vi "Save spectrum data.vi"(9 "Sample Temperature Unit":u16(ring) items=["Kelvin", "Celcius", "Sensor Units"], 10 "Data Spectrum":dbl[][](array[numeric])) -> ()   [LabVIEW 2009]
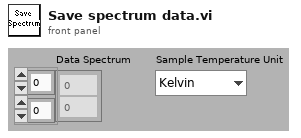
[diagram p1: front panel]
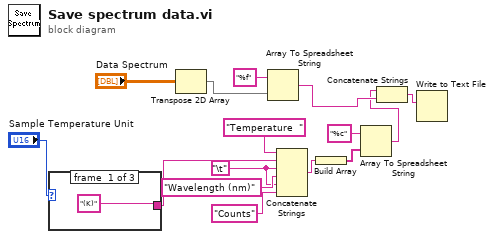
[diagram p0: block diagram]
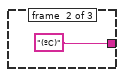
[diagram p2: hidden frame]
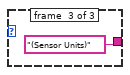
[diagram p3: hidden frame]
diagram:
  w5 = "\t"
  n1 = case shown="0, Default" "Sample Temperature Unit" {
    tunnel: ["(K)" "(ºC)" "(Sensor Units)"] -> w14
    frame #0 {
    }
    frame #1 {
    }
    frame #2 {
    }
  }
  n2 = Transpose 2D Array(2D array="Data Spectrum") -> (transposed array=w10:dbl[][])
  n3 = Array To Spreadsheet String(array=w10, 3:"%f") -> (spreadsheet string=w8:string)  [unwired: 1 in]
  n4 = Concatenate Strings("Temperature  ", w14, w5, "Wavelength (nm)", w5, "Counts") -> (w13:string)
  n5 = Build Array(w13) -> (w12:string[])
  n6 = Array To Spreadsheet String(array=w12, 3:"%c" ("format string")) -> (spreadsheet string=w3:string)  [unwired: 1 in]
  n7 = Concatenate Strings(w3, w8) -> (w7:string)
  n8 = Write to Text File(text=w7) -> ()  [unwired: 3 in, 3 out]
